vi "Read Promoted Devices.vi"() -> (0 "error out":errorcluster, 3 "promoted devices":string[](array[string]))   [LabVIEW 2024, in "Dynamic Signal Acquisition (Interactive) UI.lvlib"]
uses:
  <vilib>/Utility/config.llb/Read Key (String).vi
  Dynamic Signal Acquisition (Interactive) UI.lvlib
  <vilib>/Utility/config.llb/NI_LVConfig.lvlib
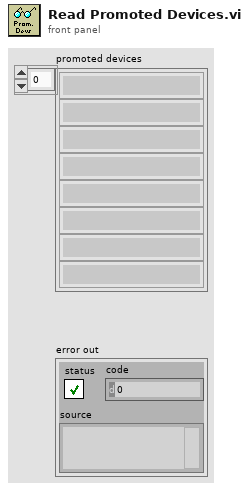
[diagram p1: front panel]
types:
  T1 = typedef "NI_LVConfig.lvlib/Config Data RefNum.ctl" = refnum<k1>
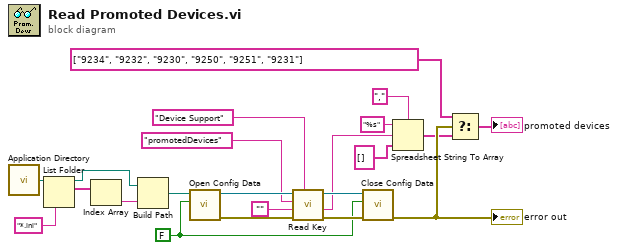
[diagram p0: block diagram]
diagram:
  w10 = FALSE ("create file if necessary (T)")
  n1 = call <vilib>:"Application Directory.vi"() -> ("Application Directory"=w16:path)
  n2 = List Folder(path=w16, pattern="*.ini") -> (path out=w13:path, filenames=w14:string[])  [unwired: 2 in, 2 out]
  n3 = Index Array(array=w14) -> (element=w12:string)  [unwired: 1 in]
  n4 = Build Path(base path=w13, name or relative path=w12) -> (appended path=w11:path)
  n5 = call <vilib>:"Open Config Data.vi"("create file if necessary (T)"=w10, "configuration file path"=w11) -> ("error out"=w21:errorcluster, "refnum"=w22:T1)  [unwired: 7 in, 1 out]
  n6 = call-poly <vilib>:"Read Key.vi"("section"="Device Support", "error in (no error)"=w21, "default value"="", "key"="promotedDevices" ("section"), "refnum"=w22) -> ("error out"=w19:errorcluster, "value"=w8:string, "refnum out"=w20:T1)  [unwired: 3 in, 1 out]
  n7 = call <vilib>:"Close Config Data.vi"("error in (no error)"=w19, "write file if changed (T)"=w10, "refnum"=w20) -> ("error out"=w4:errorcluster)  [unwired: 7 in, 1 out]
  "error out" <- w4
  n8 = Spreadsheet String To Array(delimiter (Tab)=",", format string="%s", spreadsheet string=w8, array type (2D Dbl)=string[] []) -> (array=w2:string[])
  n9 = Select(t=string[] ["9234", "9232", "9230", "9250", "9251", "9231"] ("promoted devices"), s=w4, f=w2) -> (s? t:f=→"promoted devices":string[])
